vi "CryoCon Load Calibration-new.vi"(0 "Instrument Address":refnum<visa-resource-name>, 1 "Sensor Type":T1=enum."AC Resistance", 2 "Sensor Number":u32=1 min=1 max=12 step=1, 3 "Error In":errorcluster, 4 "Calibration (Empty gives dialog)":string) -> (5 "dup VISA session":refnum<visa-resource-name>, 8 "error out":errorcluster {"code" format="%.0x"})   [LabVIEW 2019]
doc: "This VI loads a calibration file into the Conductus LTC-20 temperature controller. The file is a line of up to 19 characters of ID info, followed by the temperature information in 2 columns of temperature and resistance (sensor value)\nScott Hannahs, NHMFL-FSU, March 1995"
uses:
  Sub Controls/CryoCon Sensor Type.ctl
panel:
  out "Status":string
  out "String Read":string
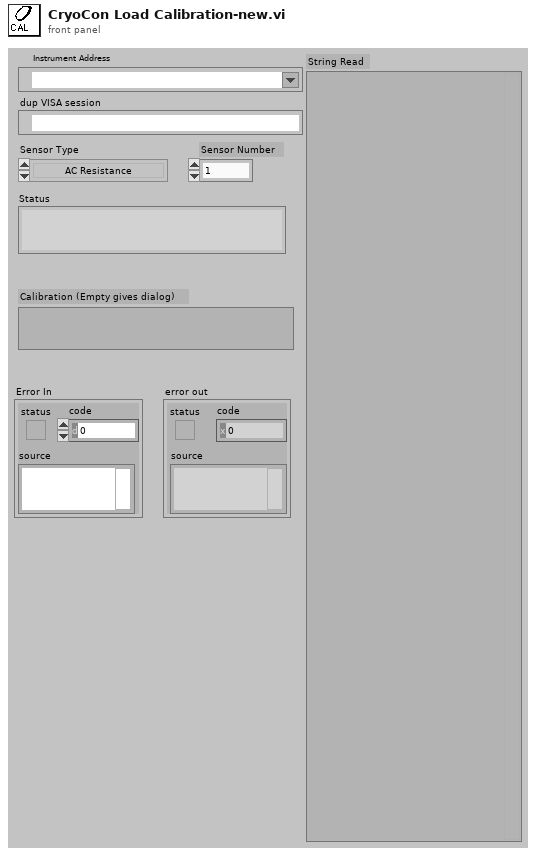
[diagram p1: front panel]
types:
  T1 = typedef "CryoCon Sensor Type.ctl" = enum16{"Diode", "AC Resistance", "DC Resistance 3.1 k½", "DC Resistance 312 ½", "DC Resistance 625 ½"}
  T2 = enum32{"Invalid", "Standard", "Closed", "Hidden", "Minimized", "Maximized"}
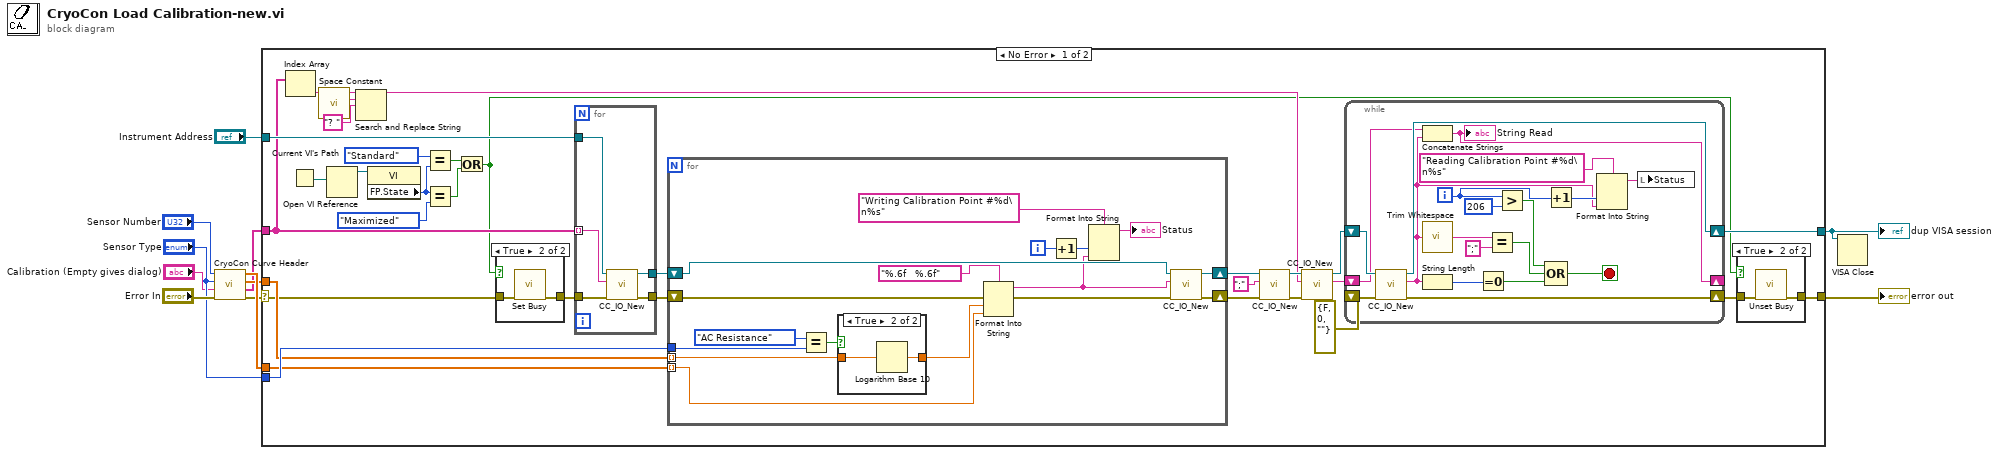
[diagram p0: block diagram]
diagram:
  n1 = call "CryoCon Curve Header.vi"("Error In"="Error In", "Calibration (Empty gives dialog)"="Calibration (Empty gives dialog)", "Sensor Type"="Sensor Type", "Sensor Number"="Sensor Number") -> ("error out"=w4:errorcluster, "Header Array"=w5:string[], "Resistance"=w8:dbl[], "Temperature"=w9:dbl[])
  n2 = case shown="No Error" w4 {
    selector: w4 -> [w33 w94]
    tunnel: w5 -> [w31 _]
    tunnel: "Sensor Type" -> [w43 _]
    tunnel: [w32 w94] -> w10
    tunnel: [w23 w95] -> w3
    tunnel: w9 -> [w39 _]
    tunnel: w8 -> [w38 _]
    tunnel: "Instrument Address" -> [w35 w95]
    frame No Error {
      n3 = Index Array(array=w31) -> (element=w21:string)  [unwired: 1 in]
      n4 = Current VI's Path() -> (path=w14:path)
      n5 = call <vilib>:"Space Constant.vi"() -> ("String"=w27:string)
      n6 = Open VI Reference(vi path=w14) -> (vi reference=w20:refnum<vi>)  [unwired: 5 in, 1 out]
      n7 = Search and Replace String(input string=w21, search string=w27, replace string="? " ("replace string (\"\")")) -> (result string=w28:string)  [unwired: 5 in, 3 out]
      n8 = property class="VI"(reference=w20) -> ("FP.State"=w17:T2)  [unwired: 1 in, 2 out]
      n9 = Equal?(x=T2."Standard" ("Front Panel Window:State"), y=w17) -> (x = y?=w16:bool)
      n10 = Equal?(x=w17, y=T2."Maximized" ("Front Panel Window:State")) -> (x = y?=w15:bool)
      n11 = Or(x=w16, y=w15) -> (x .or. y?=w13:bool)
      n12 = case shown="True" w13 {
        tunnel: [w47 w49] -> w34
        tunnel: w33 -> [w47 w48]
        frame False {
        }
        frame True {
          n13 = call <vilib>:"Set Busy.vi"("error in (no error)"=w48) -> ("error out"=w49:errorcluster)  [unwired: 9 in, 1 out]
        }
      }
      n14 = for {
        tunnel: w31 -> [w69] mode=indexing
        tunnel: w34 -> [w73]
        tunnel: [w72] -> w42
        tunnel: [w71] -> w40
        tunnel: w35 -> [w70]
        n15 = call "CC_IO_New.vi"("error in (no error)"=w73, "Command String"=w69, "VISA Refnum in"=w70) -> ("error out"=w72:errorcluster, "VISA Refnum out"=w71:refnum<visa-resource-name>)  [unwired: 6 in, 1 out]
      }
      n16 = for {
        tunnel: w43 -> [w90]
        shift-right: [w86] -> w36
        shift-left: w42 -> [w88]
        shift-right: [w87] -> w37
        shift-left: w40 -> [w85]
        tunnel: w39 -> [w80] mode=indexing
        tunnel: w38 -> [w82] mode=indexing
        i -> [w78]
        n17 = Equal?(x=CryoCon_Sensor_Type."AC Resistance" ("Sensor Type"), y=w90) -> (x = y?=w89:bool)
        n18 = case shown="True" w89 {
          tunnel: w82 -> [w91 w93]
          tunnel: [w91 w92] -> w79
          frame False {
          }
          frame True {
            n19 = Logarithm Base 10(1:w93) -> (0:w92:dbl)
          }
        }
        n20 = Format Into String(format string="%.6f   %.6f" ("Format String"), error in=w88, w79, w80) -> (resulting string=w74:string, error out=w83:errorcluster)  [unwired: 1 in]
        n21 = Increment(x=w78) -> (x+1=w77:i32)
        n22 = Format Into String(format string="Writing Calibration Point #%d\n%s", w77, w74) -> (resulting string=→"Status":string)  [unwired: 2 in, 1 out]
        n23 = call "CC_IO_New.vi"("error in (no error)"=w83, "Command String"=w74, "VISA Refnum in"=w85) -> ("error out"=w86:errorcluster, "VISA Refnum out"=w87:refnum<visa-resource-name>)  [unwired: 6 in, 1 out]
      }
      n24 = call "CC_IO_New.vi"("error in (no error)"=w36, "Command String"=";", "VISA Refnum in"=w37) -> ("error out"=w29:errorcluster, "VISA Refnum out"=w30:refnum<visa-resource-name>)  [unwired: 6 in, 1 out]
      n25 = call "CC_IO_New.vi"("error in (no error)"=w29, "Command String"=w28, "VISA Refnum in"=w30) -> ("String Read"=w22:string, "VISA Refnum out"=w24:refnum<visa-resource-name>)  [unwired: 6 in, 1 out]
      n26 = while {
        shift-right: [w52] -> _
        shift-left: w22 -> [w64]
        shift-right: [w67] -> w25
        shift-left: errorcluster {"status"=FALSE, "code"=0, "source"=""} ("error out") -> [w68]
        shift-right: [w65] -> w23
        shift-left: w24 -> [w66]
        i -> [w57]
        stop <- w60 stop-if-true
        n27 = call "CC_IO_New.vi"("error in (no error)"=w68, "VISA Refnum in"=w66) -> ("error out"=w67:errorcluster, "String Read"=w50:string, "VISA Refnum out"=w65:refnum<visa-resource-name>)  [unwired: 7 in]
        n28 = Concatenate Strings(w64, w50) -> (w52:string)
        "String Read" <- w52
        n29 = call <vilib>:"Trim Whitespace.vi"("string"=w50) -> ("trimmed string"=w51:string)  [unwired: 1 in]
        n30 = String Length(string=w50) -> (length=w54:i32)
        n31 = Equal To 0?(x=w54) -> (x = 0?=w53:bool)
        n32 = Equal?(x=w51, y=";") -> (x = y?=w61:bool)
        n33 = Greater?(x=w57, y=206) -> (0:w55:bool)
        n34 = Compound Arithmetic op=OR(w55, w61, w53) -> (w60:bool)
        n35 = Increment(x=w57) -> (x+1=w59:i32)
        n36 = Format Into String(format string="Reading Calibration Point #%d\n%s", w59, w50) -> (resulting string=w56:string)  [unwired: 2 in, 1 out]
        n37 = local write "Status"(w56) -> ()
      }
      n38 = case shown="True" w13 {
        tunnel: [w44 w46] -> w32
        tunnel: w25 -> [w44 w45]
        frame False {
        }
        frame True {
          n39 = call <vilib>:"Unset Busy.vi"("error in (no error)"=w45) -> ("error out"=w46:errorcluster)  [unwired: 10 in]
        }
      }
    }
    frame Error {
    }
  }
  "dup VISA session" <- w3
  "error out" <- w10
  n40 = VISA Close(VISA resource name=w3) -> ()  [unwired: 1 in, 1 out]
